vi "GT Get Var Calculate.vi"(8 "error in (no error)":errorcluster caption="错误输入（无错误）", 9 "pVarCalculate":T1, 10 "index":i16, 11 "cardNum":i16) -> (0 "error out":errorcluster caption="错误输出", 1 "pVarCalculate out":T1, 3 "function return":i16)   [LabVIEW 2020, in "gts1.lvlib"]
doc: "GT_API GT_GetVarCalculate(short cardNum,short index,TVarCalculate *pVarCalculate);"
uses:
  gts1.lvlib
  dll/32bit/multi_card/gts.dll
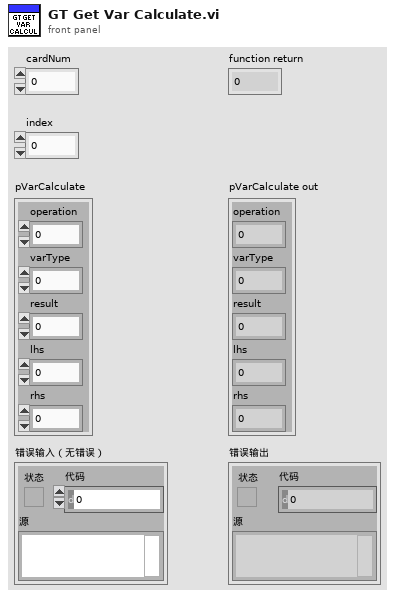
[diagram p1: front panel]
types:
  T1 = cluster{"operation":u16, "varType":u16, "result":u16, "lhs":u16, "rhs":u16}
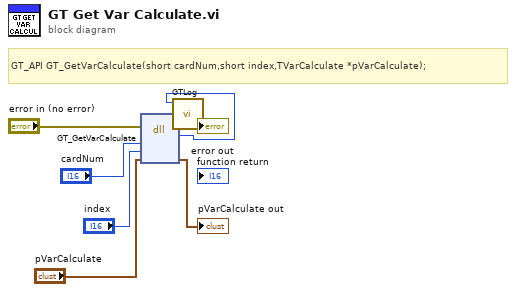
[diagram p0: block diagram]
diagram:
  # "GT_API GT_GetVarCalculate(short cardNum,short index,TVarCalculate *pVarCalculate);"
  n1 = dll-call lib="C:/1228/dll/32bit/multi_card/gts.dll" fn="GT_GetVarCalculate"(error in="error in (no error)", "cardNum"="cardNum", "index"="index", "pVarCalculate"="pVarCalculate") -> (error out=w3:errorcluster, w1:i16, "pVarCalculate"=→"pVarCalculate out":T1)  [unwired: 4 in, 1 out]
  n2 = call "GTLog.vi"("error in (no error)"=w3, "Numeric"=w1) -> ("error out"=→"error out":errorcluster)  [unwired: 9 in]
